vi "Init.vi"(8 "error in (no error)":errorcluster, 10 "Shutdown Event":refnum<user-event>, 11 "Controller Interface in":refnum<class "Controller Interface.lvclass">) -> (0 "error out":errorcluster, 3 "Controller Interface out":refnum<class "Controller Interface.lvclass">)   [LabVIEW 2019, in "Controller Interface.lvlib" / "Controller Interface.lvclass"]
uses:
  Controller Interface.lvclass
  Controller Interface.lvclass/Controller Interface.ctl
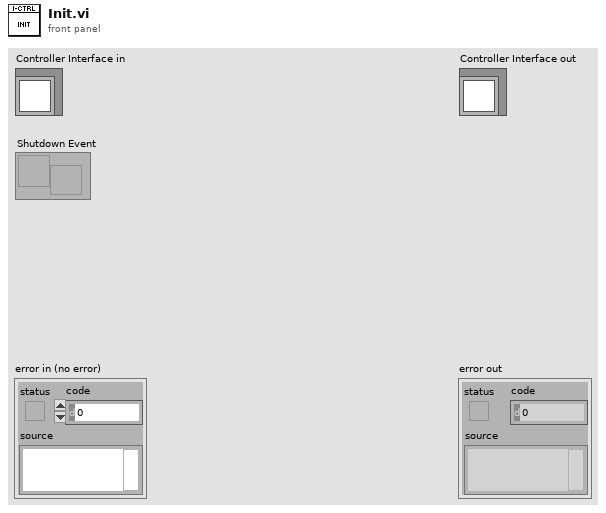
[diagram p1: front panel]
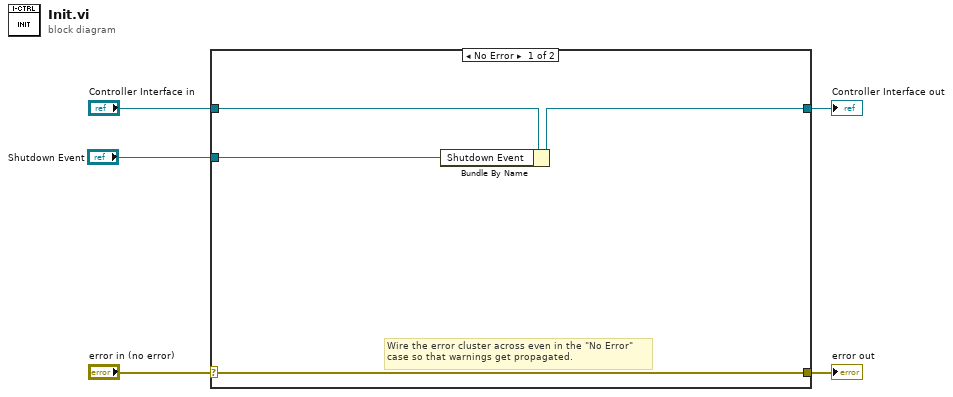
[diagram p0: block diagram]
diagram:
  n1 = case shown="No Error" "error in (no error)" {
    selector: "error in (no error)" -> [w9 w11]
    tunnel: [w9 w11] -> w4
    tunnel: [w7 w10] -> w2
    tunnel: "Controller Interface in" -> [w6 w10]
    tunnel: "Shutdown Event" -> [w8 _]
    frame No Error {
      # "Wire the error cluster across even in the \"No Error\"\ncase so that warnings get propagated."
      n2 = Bundle By Name(cluster=w6, "Shutdown Event"=w8) -> (w7:refnum<class "Controller Interface.lvclass">)
    }
    frame Error {
    }
  }
  "error out" <- w4
  "Controller Interface out" <- w2
